vi "read.vi"(8 "error in":errorcluster, 11 "Text Session in":refnum<class "FPGA Serial Session.lvclass">) -> (0 "error out":errorcluster, 2 "Data Out":string, 3 "Text Session out":refnum<class "FPGA Serial Session.lvclass">)   [LabVIEW 2015, in "FPGA Serial Session.lvclass"]
uses:
  FPGA Serial Session.lvclass
  FPGA Serial Session.lvclass/FPGA Serial Session.ctl
  Raw FPGA/FPGA Session.lvclass
  FPGA/Serial Data In.ctl
  Raw FPGA/FPGA Session.lvclass/FPGA Session.ctl
  Raw FPGA/Read FPGA Ref.vi
  <vilib>/rvi/errors/niLvFpgaAdjustHostInterfaceError.vi
  <vilib>/Utility/error.llb/Error Cluster From Error Code.vi
  <vilib>/RVI Host/nirviSupport.llb/nirviErrorClusterFromErrorCode.vi
  FPGA Ref.ctl
  FPGA/RS485 In.ctl
  <vilib>/rvi/interface/nirviReadWriteControl/nirviReadWriteControl.xnode
  FPGA Bitfiles/NickIO.lvbitx
  <vilib>/rvi/interface/nirviMethod/nirviMethod.xnode
  NiFpgaLv.dll
  <vilib>/FPGAPlugInAG/cRIO-9081/niLvFpga_AcknowledgeIrq_cRIO-9081.vi
  <vilib>/rvi/interface/nirviMethod/StockFPGA_InlinedMethodWaitForSingleIRQ.vi
  <vilib>/FPGAPlugInAG/cRIO-9081/niLvFpga_WaitOnIrq_cRIO-9081.vi
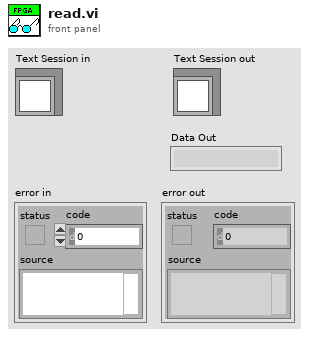
[diagram p1: front panel]
types:
  T1 = typedef "Serial Data In.ctl" = cluster{"Data":u8[], "NumBytes":i32, "RS485_Cmd":enum8{"Read", "Write", "Idle"}, "Timeout (ms)":i32}
  T2 = typedef "Session - Root.lvclass/Session Handle.ctl" = refnum<data-value>
  T3 = enum16{"Port 1", "Port 2", "Port 3", "Port 4", "None"}
  T4 = typedef "FPGA Ref.ctl" = refnum<k20>
  T5 = typedef "RS485 In.ctl" = cluster{"Data":u8[], "NumBytes":i32, "New":bool}
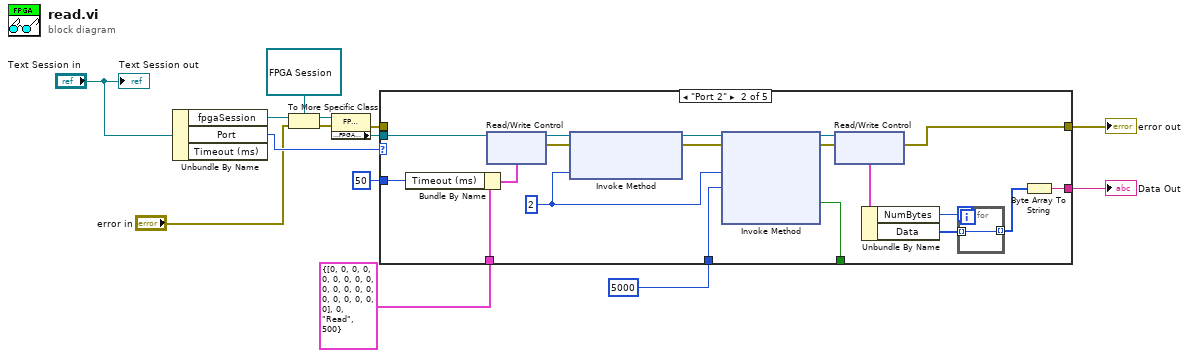
[diagram p0: block diagram]
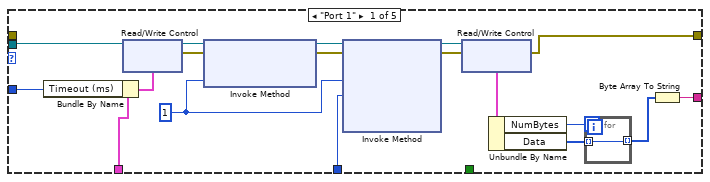
[diagram p2: hidden frame]
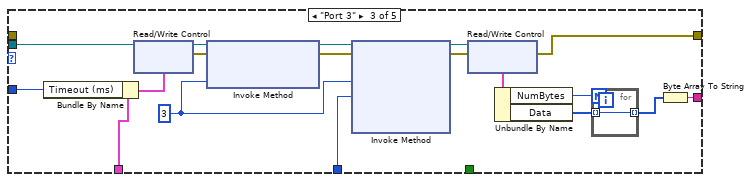
[diagram p3: hidden frame]
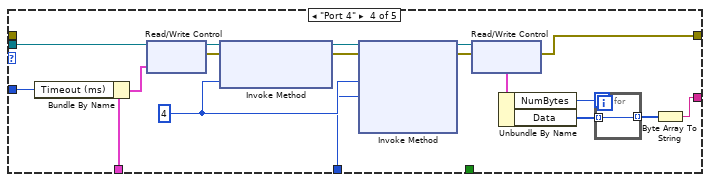
[diagram p4: hidden frame]
diagram:
  n1 = Unbundle By Name("Text Session in") -> ("fpgaSession"=w12:T2, "Port"=w13:T3)  [unwired: 1 out]
  n2 = To More Specific Class(target class=refnum<data-value> refnum, reference=w12, error in="error in") -> (specific class reference=w10:refnum<data-value>, error out=w7:errorcluster)
  n3 = property class="FPGA Session"(reference=w10, error in=w7) -> (error out=w6:errorcluster, "Accessors:FPGA Ref"=w9:T4)  [unwired: 1 out]
  n4 = case shown="\"Port 2\"" w13 {
    tunnel: w9 -> [w23 w52 w71 w90 _]
    tunnel: w6 -> [_ _ _ _ w92]
    tunnel: [w21 w43 w61 w82 _] -> w5
    tunnel: [w22 w42 w60 w81 w92] -> w4
    tunnel: 5000 ("Timeout (ms)") -> [w20 w41 w59 w80 _]
    tunnel: 50 ("Timeout (ms)") -> [w16 w36 w55 w75 _]
    tunnel: T1 {"Data"=[0, 0, 0, 0, 0, 0, 0, 0, 0, 0, 0, 0, 0, 0, 0, 0, 0, 0, 0, 0], "NumBytes"=0, "RS485_Cmd"=enum."Read", "Timeout (ms)"=500} ("Port4 In") -> [w15 w35 w54 w73 _]
    tunnel: [_ w34 _ _ _] -> _
    frame "Port 1" {
      w27 = 1 ("IRQ Number(s)")
      n5 = Bundle By Name(cluster=w15, "Timeout (ms)"=w16) -> (w32:T1)
      n6 = xnode "Read/Write Control"("FPGA VI Reference In"=w23, "Port1 In"=w32) -> ("FPGA VI Reference Out"=w29:T4, "error out"=w28:errorcluster)  [unwired: 1 in]
      n7 = xnode "Invoke Method"("FPGA VI Reference In"=w29, "error in"=w28, "IRQ Number(s)"=w27) -> ("FPGA VI Reference Out"=w31:T4, "error out"=w30:errorcluster)
      n8 = xnode "Invoke Method"("FPGA VI Reference In"=w31, "error in"=w30, "IRQ Number(s)"=w27, "Timeout (ms)"=w20) -> ("FPGA VI Reference Out"=w26:T4, "error out"=w25:errorcluster)  [unwired: 2 out]
      n9 = xnode "Read/Write Control"("FPGA VI Reference In"=w26, "error in"=w25) -> ("error out"=w22:errorcluster, "Port1 Out"=w24:T5)  [unwired: 1 out]
      n10 = Unbundle By Name(w24) -> ("NumBytes"=w19:i32, "Data"=w18:u8[])
      n11 = for {
        N: w19 -> [_]
        tunnel: w18 -> [w33] mode=indexing
        tunnel: [w33] -> w17 mode=indexing
      }
      n12 = Byte Array To String(unsigned byte array=w17) -> (string=w21:string)
    }
    frame "Port 2" {
      w46 = 2 ("IRQ Number(s)")
      n13 = Bundle By Name(cluster=w35, "Timeout (ms)"=w36) -> (w51:T1)
      n14 = xnode "Read/Write Control"("FPGA VI Reference In"=w52, "Port2 In"=w51) -> ("FPGA VI Reference Out"=w48:T4, "error out"=w47:errorcluster)  [unwired: 1 in]
      n15 = xnode "Invoke Method"("FPGA VI Reference In"=w48, "error in"=w47, "IRQ Number(s)"=w46) -> ("FPGA VI Reference Out"=w50:T4, "error out"=w49:errorcluster)
      n16 = xnode "Invoke Method"("FPGA VI Reference In"=w50, "error in"=w49, "IRQ Number(s)"=w46, "Timeout (ms)"=w41) -> ("FPGA VI Reference Out"=w45:T4, "error out"=w44:errorcluster, "Timed Out"=w34:bool)  [unwired: 1 out]
      n17 = xnode "Read/Write Control"("FPGA VI Reference In"=w45, "error in"=w44) -> ("error out"=w42:errorcluster, "Port2 Out"=w38:T5)  [unwired: 1 out]
      n18 = Unbundle By Name(w38) -> ("NumBytes"=w40:i32, "Data"=w39:u8[])
      n19 = for {
        N: w40 -> [_]
        tunnel: w39 -> [w53] mode=indexing
        tunnel: [w53] -> w37 mode=indexing
      }
      n20 = Byte Array To String(unsigned byte array=w37) -> (string=w43:string)
    }
    frame "Port 3" {
      w65 = 3 ("IRQ Number(s)")
      n21 = Bundle By Name(cluster=w54, "Timeout (ms)"=w55) -> (w70:T1)
      n22 = xnode "Read/Write Control"("FPGA VI Reference In"=w71, "Port3 In"=w70) -> ("FPGA VI Reference Out"=w67:T4, "error out"=w66:errorcluster)  [unwired: 1 in]
      n23 = xnode "Invoke Method"("FPGA VI Reference In"=w67, "error in"=w66, "IRQ Number(s)"=w65) -> ("FPGA VI Reference Out"=w69:T4, "error out"=w68:errorcluster)
      n24 = xnode "Invoke Method"("FPGA VI Reference In"=w69, "error in"=w68, "IRQ Number(s)"=w65, "Timeout (ms)"=w59) -> ("FPGA VI Reference Out"=w64:T4, "error out"=w63:errorcluster)  [unwired: 2 out]
      n25 = xnode "Read/Write Control"("FPGA VI Reference In"=w64, "error in"=w63) -> ("error out"=w60:errorcluster, "Port3 Out"=w62:T5)  [unwired: 1 out]
      n26 = Unbundle By Name(w62) -> ("NumBytes"=w58:i32, "Data"=w57:u8[])
      n27 = for {
        N: w58 -> [_]
        tunnel: w57 -> [w72] mode=indexing
        tunnel: [w72] -> w56 mode=indexing
      }
      n28 = Byte Array To String(unsigned byte array=w56) -> (string=w61:string)
    }
    frame "Port 4" {
      w85 = 4 ("IRQ Number(s)")
      n29 = Bundle By Name(cluster=w73, "Timeout (ms)"=w75) -> (w74:T1)
      n30 = xnode "Read/Write Control"("FPGA VI Reference In"=w90, "Port4 In"=w74) -> ("FPGA VI Reference Out"=w87:T4, "error out"=w86:errorcluster)  [unwired: 1 in]
      n31 = xnode "Invoke Method"("FPGA VI Reference In"=w87, "error in"=w86, "IRQ Number(s)"=w85) -> ("FPGA VI Reference Out"=w89:T4, "error out"=w88:errorcluster)
      n32 = xnode "Invoke Method"("FPGA VI Reference In"=w89, "error in"=w88, "IRQ Number(s)"=w85, "Timeout (ms)"=w80) -> ("FPGA VI Reference Out"=w84:T4, "error out"=w83:errorcluster)  [unwired: 2 out]
      n33 = xnode "Read/Write Control"("FPGA VI Reference In"=w84, "error in"=w83) -> ("error out"=w81:errorcluster, "Port4 Out"=w77:T5)  [unwired: 1 out]
      n34 = Unbundle By Name(w77) -> ("NumBytes"=w79:i32, "Data"=w78:u8[])
      n35 = for {
        N: w79 -> [_]
        tunnel: w78 -> [w91] mode=indexing
        tunnel: [w91] -> w76 mode=indexing
      }
      n36 = Byte Array To String(unsigned byte array=w76) -> (string=w82:string)
    }
    frame "None", Default {
    }
  }
  "error out" <- w4
  "Data Out" <- w5
  "Text Session out" <- "Text Session in"
